vi "myRIO_BRig_RT__Case_Exp__recordLick.vi"(4 "intput_state__trialEnd":T1, 6 "intput_state__trialStart":T1, 8 "input_lick__R":bool, 9 "input_lick__L":bool, 10 "input_dataCurrent":u16[](array[numeric]), 11 "input_dataLick":u16[][](array[numeric])) -> (2 "output_dataCurrent":u16[](array[numeric]), 3 "output_dataLick":u16[][](array[numeric]))   [LabVIEW 2014]
uses:
  myRIO_BRig_RT__Case_Exp_stateList.ctl
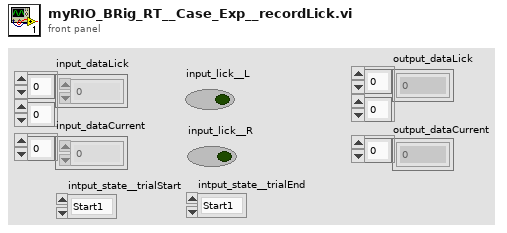
[diagram p1: front panel]
types:
  T1 = typedef "myRIO_BRig_RT__Case_Exp_stateList.ctl" = enum16{"Start1", "Start2", "Start3", "saveSettings1", "saveSettings2", "saveSettings3", "saveSettings4", "saveSettings_LC_ENL_l1", "saveSettings_LC_ENL_l2", "saveSettings_LC_Cue_l1", "saveSettings_LC_Cue_l2", "saveSettings6_LC_l1_Other", "SaveSettings6_LC_l2_Other", "setSettings_Audio", "setSettings_Laser", "initBlock_pre", "initBlock", "initBlock2", "initBlock_post", "initTrial_pre", "initTrial", "initTrial2", "initTrial3", "initTrial4", "initTrial_LC_ENL1", "initTrial_LC_Cue1", "initTrial_LC_Cue1_2", "initTrial_LC_Sel", "initTrial_post", "ENL1_pre", "ENL1", "ENL1_post", "ENL1Penalty_pre", "ENL1Penalty", "ENL2_pre", "ENL2", "ENL2Penalty_pre", "ENL2Penalty", "Cue1_pre", "Cue1", "Cue1_post", "Cue1Penalty_pre", "Cue1Penalty", "Cue2_pre", "Cue2", "Cue2Penalty_pre", "Cue2Penalty", "Selection_pre", "Selection", "Select_post", "SelectReward_pre", "SelectReward", "SelectRewardPost_pre", "SelectRewardPost", "SelectWrong_pre", "SelectWrong", "SelectWrong_post", "SelectTimeout_pre", "SelectTimeout", "SelectTimeout_post", "endTrial_pre", "endTrial1", "endTrial2", "endTrial3", "endTrial_post", "endBlock_pre", "endBlock", "endBlock_post", "endExp", "commConnect", "commUpload_pre", "commUpload_dataBlock", "commUpload_dataCurrent", "commUpload_dataExp", "commUpload_dataLC", "commUpload_dataTrial", "commUpload_post", "saveData_pre", "saveData_dataBlock", "saveData_dataCurrent", "saveData_dataExp", "saveData_dataLC", "saveData_dataTrial", "saveData_post", "empty_endBlock1", "empty_endBlock2", "empty_endTrial1", "empty_endTrial2", "empty_endTrial3", "empty_endTrial4", "empty_endTrial5", "dummyState", "dummyState_endBlock"}
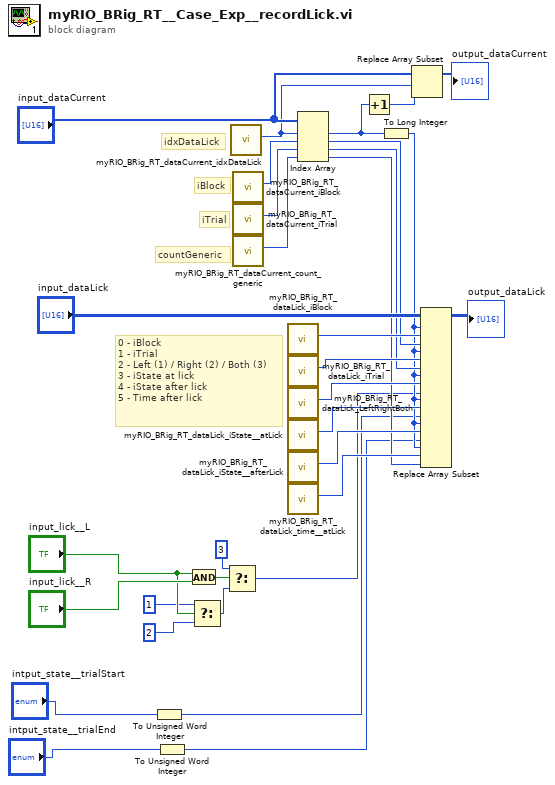
[diagram p0: block diagram]
diagram:
  # "0 - iBlock\n1 - iTrial\n2 - Left (1) / Right (2) / Both (3)\n3 - iState at lick\n4 - iState after lick\n5 - Time after lick"
  # "idxDataLick"
  # "countGeneric"
  # "iTrial"
  # "iBlock"
  n1 = To Unsigned Word Integer(number="intput_state__trialStart") -> (unsigned 16bit integer=w4:u16)
  n2 = To Unsigned Word Integer(number="intput_state__trialEnd") -> (unsigned 16bit integer=w3:u16)
  n3 = And(x="input_lick__L", y="input_lick__R") -> (x .and. y?=w14:bool)
  n4 = Select(t=u16 1, s="input_lick__L", f=u16 2) -> (s? t:f=w6:u16)
  n5 = Select(t=u16 3, s=w14, f=w6) -> (s? t:f=w5:u16)
  n6 = call "myRIO_BRig_RT_dataCurrent_idxDataLick.vi"() -> ("output_idxDataLick"=w26:i32)  [unwired: 11 in]
  n7 = call "myRIO_BRig_RT_dataCurrent_iBlock.vi"() -> ("output_iBlock"=w28:i32)  [unwired: 11 in]
  n8 = call "myRIO_BRig_RT_dataCurrent_iTrial.vi"() -> ("output_iTrial"=w29:i32)  [unwired: 11 in]
  n9 = call "myRIO_BRig_RT_dataCurrent_count_generic.vi"() -> ("output_count_generic"=w30:i32)  [unwired: 11 in]
  n10 = call "myRIO_BRig_RT_dataLick_iBlock.vi"() -> ("output_iBlock"=w23:i32)  [unwired: 11 in]
  n11 = call "myRIO_BRig_RT_dataLick_iTrial.vi"() -> ("output_iTrial"=w21:i32)  [unwired: 11 in]
  n12 = call "myRIO_BRig_RT_dataLick_LeftRightBoth.vi"() -> ("output_LeftRightBoth"=w19:i32)  [unwired: 11 in]
  n13 = call "myRIO_BRig_RT_dataLick_iState__atLick.vi"() -> ("output_iState__atLick"=w18:i32)  [unwired: 11 in]
  n14 = call "myRIO_BRig_RT_dataLick_iState__afterLick.vi"() -> ("output_iState__afterLick"=w17:i32)  [unwired: 11 in]
  n15 = call "myRIO_BRig_RT_dataLick_time__atLick.vi"() -> ("output_time__atLick"=w16:i32)  [unwired: 11 in]
  n16 = Index Array(array="input_dataCurrent", index #1=w26, index #2=w28, index #3=w29, index #4=w30) -> (element #1=w13:u16, element #2=w22:u16, element #3=w20:u16, element #4=w15:u16)
  n17 = Increment(x=w13) -> (x+1=w25:u16)
  n18 = To Long Integer(number=w13) -> (32bit integer=w12:i32)
  n19 = Replace Array Subset(array="input_dataCurrent", new element=w25, index=w26) -> (→"output_dataCurrent":u16[])
  n20 = Replace Array Subset(array="input_dataLick", new element #1=w22, index (row) #1=w12, index (col) #1=w23, new element #2=w20, index (row) #2=w12, index (col) #2=w21, new element #3=w5, index (row) #3=w12, index (col) #3=w19, new element #4=w4, index (row) #4=w12, index (col) #4=w18, new element #5=w3, index (row) #5=w12, index (col) #5=w17, new element #6=w15, index (row) #6=w12, index (col) #6=w16) -> (→"output_dataLick":u16[][])
